vi "test queue.vi"() -> ()   [LabVIEW 2019]
uses:
  Controls/FGV States.ctl
panel:
  out "timed out?":bool
  out "error out 3":errorcluster
  out "error out 2":errorcluster
  out "error out":errorcluster
  out "3":bool
  out "2":bool
  out "1":bool
  in  "stop":bool
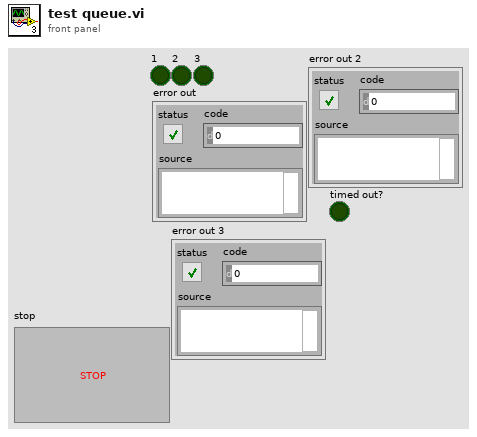
[diagram p1: front panel]
types:
  T1 = typedef "FGV States.ctl" = enum16{"Read", "Write"}
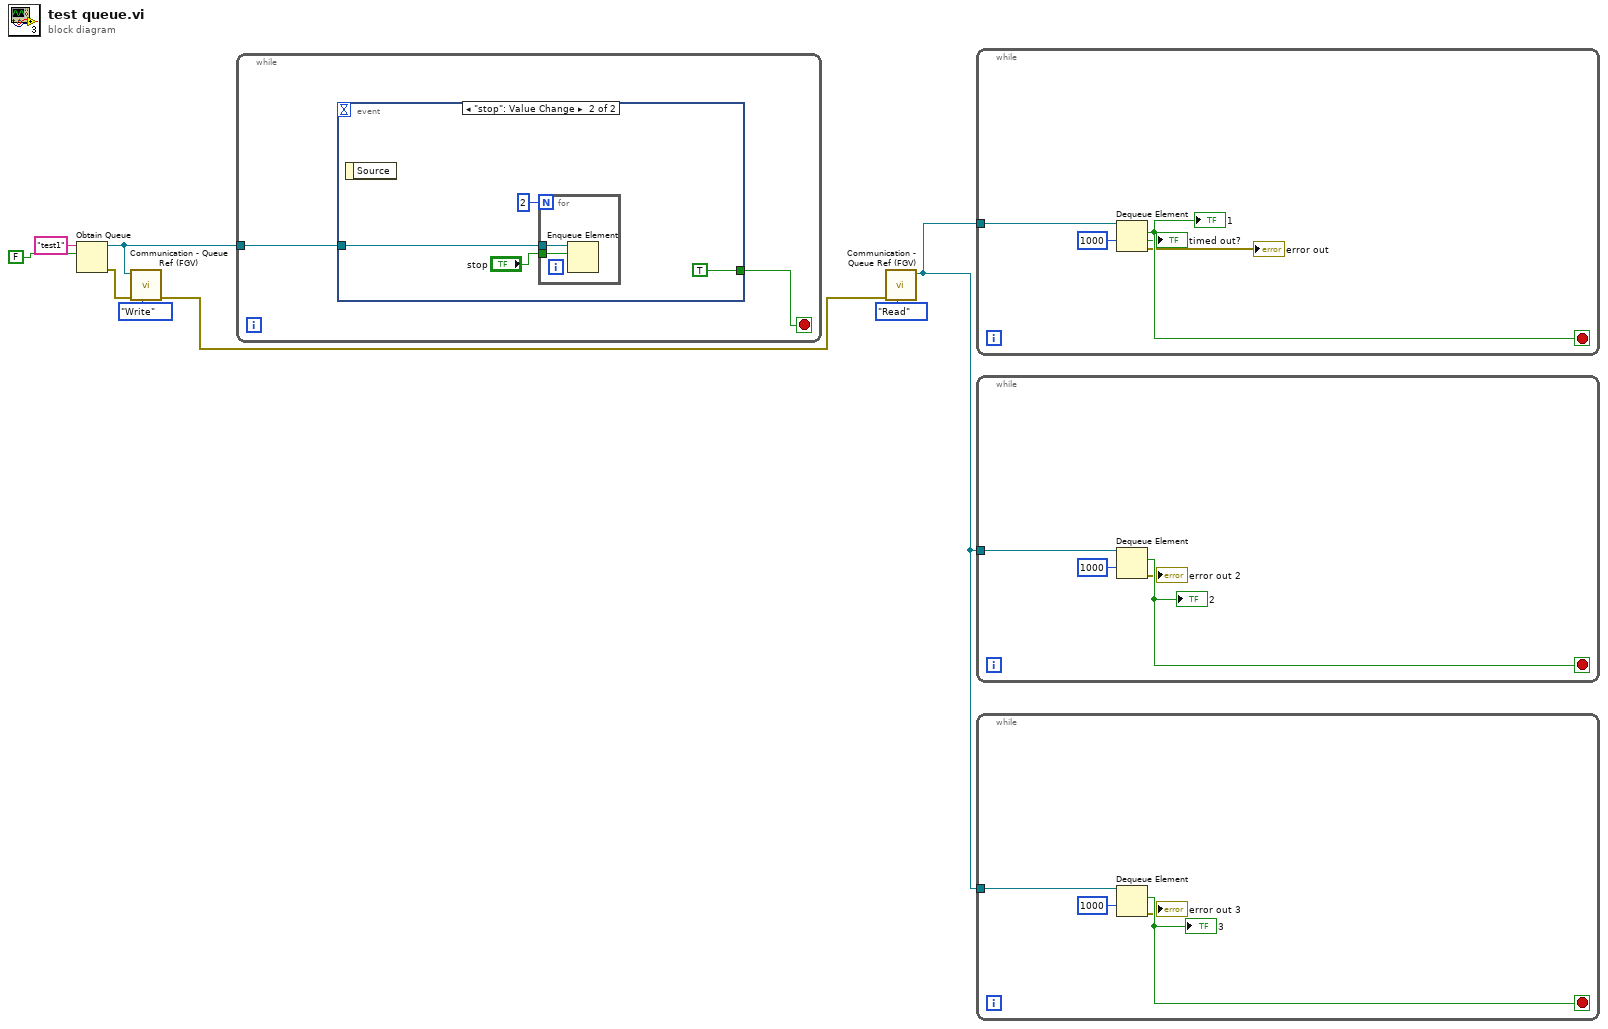
[diagram p0: block diagram]
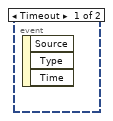
[diagram p2: hidden frame]
diagram:
  n1 = Obtain Queue(name (unnamed)="test1", element data type=FALSE) -> (queue out=w5:refnum<queue>, error out=w6:errorcluster)  [unwired: 3 in, 1 out]
  n2 = call "Communication - Queue Ref (FGV).vi"("Action"=FGV_States."Write", "error in (no error)"=w6, "queue In"=w5) -> ("error out"=w2:errorcluster)  [unwired: 7 in, 1 out]
  n3 = while {
    tunnel: w5 -> [w10]
    stop <- w9 stop-if-true
    n4 = event shown="[1] \"stop\": Value Change" {
      selector: _ -> [_ _]
      dyn-events: _ -> [_ _]
      timeout: _ -> [_ _]
      tunnel: w10 -> [_ w13]
      tunnel: [_ TRUE] -> w9
      event Timeout {
        n5 = event-data() -> ()  [unwired: 1 in, 3 out]
      }
      event "stop": Value Change {
        n6 = event-data() -> ()  [unwired: 1 in, 1 out]
        n7 = for {
          N: 2 -> [_]
          tunnel: "stop" -> [w16]
          tunnel: w13 -> [w15]
          n8 = Enqueue Element(queue=w15, element=w16) -> ()  [unwired: 2 in, 3 out]
        }
      }
    }
  }
  n9 = call "Communication - Queue Ref (FGV).vi"("Action"=FGV_States."Read", "error in (no error)"=w2) -> ("queue Out"=w1:refnum<queue>)  [unwired: 8 in, 1 out]
  n10 = while {
    tunnel: w1 -> [w21]
    stop <- w20 stop-if-true
    n11 = Dequeue Element(queue=w21, timeout in ms (-1)=1000) -> (element=w20:bool, timed out?=→"timed out?":bool, error out=→"error out":errorcluster)  [unwired: 1 in, 1 out]
    "1" <- w20
  }
  n12 = while {
    tunnel: w1 -> [w25]
    stop <- w24 stop-if-true
    n13 = Dequeue Element(queue=w25, timeout in ms (-1)=1000) -> (element=w24:bool, error out=→"error out 2":errorcluster)  [unwired: 1 in, 2 out]
    "2" <- w24
  }
  n14 = while {
    tunnel: w1 -> [w29]
    stop <- w28 stop-if-true
    n15 = Dequeue Element(queue=w29, timeout in ms (-1)=1000) -> (element=w28:bool, error out=→"error out 3":errorcluster)  [unwired: 1 in, 2 out]
    "3" <- w28
  }
